vi "VNARP-Connexion.vi"(3 "IP RP":string="169.254.8.94") -> (0 "sortie d'erreur":errorcluster, 1 "ID de connexion":refnum<k5>)   [LabVIEW 2021]
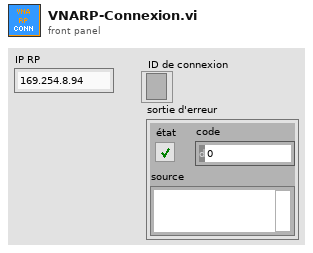
[diagram p1: front panel]
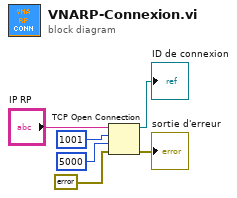
[diagram p0: block diagram]
diagram:
  n1 = TCP Open Connection(address="IP RP", remote port or service name=u16 1001 ("port distant ou nom du service"), timeout ms (60000)=5000 ("timeout en ms (60000)"), error in (no error)=errorcluster {"status"=FALSE, "code"=0, "source"=""} ("entrée d'erreur (pas d'erreur)")) -> (connection ID=→"ID de connexion":refnum<k5>, error out=→"sortie d'erreur":errorcluster)  [unwired: 1 in]
